vi "SpanConfig.vi"(8 "error in (no error)":errorcluster, 9 "Span (Hz)":dbl, 10 "Center Frequency (Hz)":dbl, 11 "SpecA_ESA in":refnum<class "SpecA_ESA.lvclass">) -> (0 "error out":errorcluster, 3 "SpecA_ESA out":refnum<class "SpecA_ESA.lvclass">)   [LabVIEW 2014, in "SpecA_ESA.lvclass"]
uses:
  SpecA_ESA.lvclass
  SpecA_ESA.lvclass/SpecA_ESA.ctl
  data/Agilent ESA PSA Series/Configure Frequency (Center Span).vi
  data/Agilent ESA PSA Series.lvlib
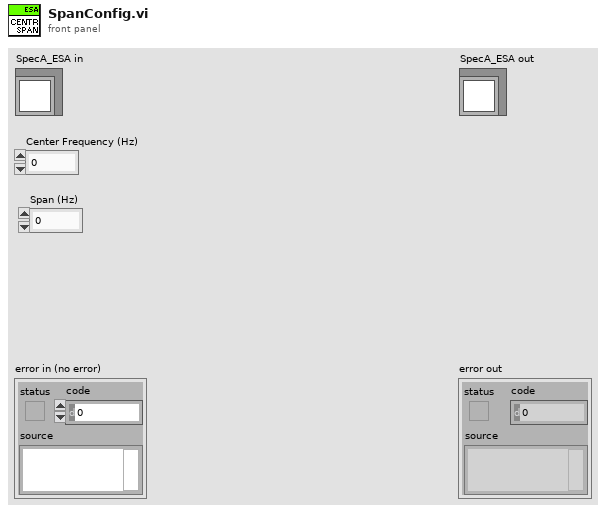
[diagram p1: front panel]
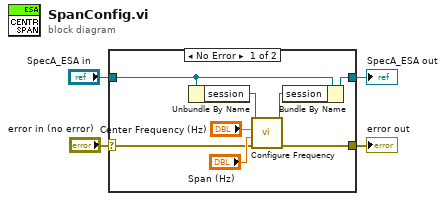
[diagram p0: block diagram]
diagram:
  n1 = case shown="No Error" "error in (no error)" {
    selector: "error in (no error)" -> [w7 w14]
    tunnel: "SpecA_ESA in" -> [w12 w13]
    tunnel: [w6 w14] -> w2
    tunnel: [w5 w13] -> w1
    frame No Error {
      n2 = Unbundle By Name(w12) -> ("session"=w11:refnum<visa-resource-name>)
      n3 = call-poly "Configure Frequency.vi"("error in (no error)"=w7, "Span (2 GHz)"="Span (Hz)", "Center Frequency (2 GHz)"="Center Frequency (Hz)", "VISA resource name"=w11) -> ("error out"=w6:errorcluster, "VISA resource name out"=w10:refnum<visa-resource-name>)  [unwired: 6 in]
      n4 = Bundle By Name(cluster=w12, "session"=w10) -> (w5:refnum<class "SpecA_ESA.lvclass">)
    }
    frame Error {
    }
  }
  "error out" <- w2
  "SpecA_ESA out" <- w1
